vi "updateDisplay.vi"(10 "display refs":T2, 11 "data":T1) -> (3 "data (dup)":T1)   [LabVIEW 2017, in "UI_TimeSelector.xctl"]
uses:
  UI_TimeSelector.xctl
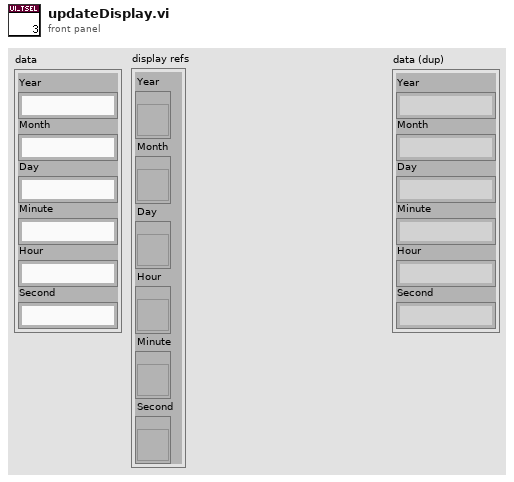
[diagram p1: front panel]
types:
  T1 = cluster{"Year":string, "Month":string, "Day":string, "Minute":string, "Hour":string, "Second":string}
  T2 = cluster{"Year":refnum<vi>, "Month":refnum<vi>, "Day":refnum<vi>, "Hour":refnum<vi>, "Minute":refnum<vi>, "Second":refnum<vi>}
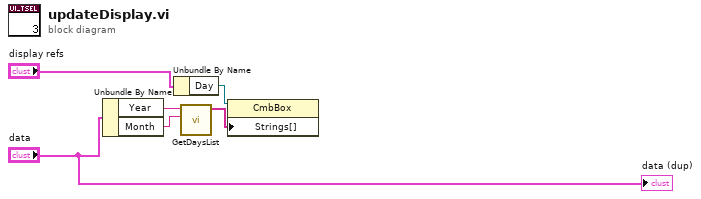
[diagram p0: block diagram]
diagram:
  n1 = Unbundle By Name("data") -> ("Year"=w4:string, "Month"=w3:string)
  n2 = Unbundle By Name("display refs") -> ("Day"=w2:refnum<vi>)
  n3 = call "GetDaysList.vi"("month"=w3, "year"=w4) -> ("Array"=w1:string[])  [unwired: 9 in]
  n4 = property class="CmbBox"(reference=w2, "Strings[]"=w1) -> ()  [unwired: 1 in, 2 out]
  "data (dup)" <- "data"
